vi "Data Buffer Status.vi"(0 "VISA resource name":refnum<visa-resource-name>, 11 "error in (no error)":errorcluster) -> (4 "VISA resource name out":refnum<visa-resource-name>, 6 "Bytes Available":i32, 8 "Bytes in Use":i32, 10 "Next Buffer Location":i32, 15 "error out":errorcluster)   [LabVIEW 2020, in "Keithley 27XX.lvlib"]
doc: "This VI returns information about the status of the buffer including Bytes Available, Bytes in Use, and Next Buffer Location."
uses:
  Keithley 27XX.lvlib
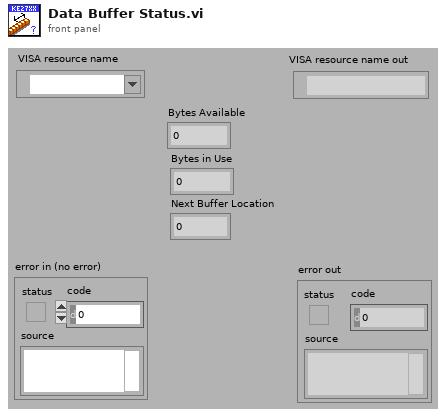
[diagram p1: front panel]
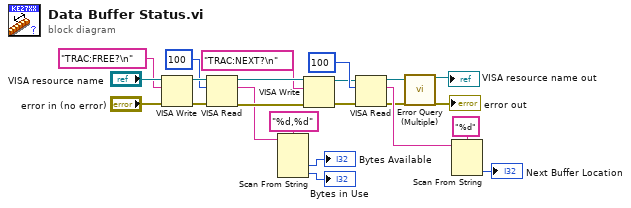
[diagram p0: block diagram]
diagram:
  n1 = VISA Write(VISA resource name="VISA resource name", write buffer="TRAC:FREE?\n", error in (no error)="error in (no error)") -> (VISA resource name out=w19:refnum<visa-resource-name>, error out=w20:errorcluster)  [unwired: 1 out]
  n2 = VISA Read(VISA resource name=w19, byte count=u32 100, error in (no error)=w20) -> (VISA resource name out=w17:refnum<visa-resource-name>, read buffer=w10:string, error out=w16:errorcluster)  [unwired: 1 out]
  n3 = Scan From String(format string="%d,%d", input string=w10) -> (output 1=→"Bytes Available":i32, output 2=→"Bytes in Use":i32)  [unwired: 4 in, 3 out]
  n4 = VISA Write(VISA resource name=w17, write buffer="TRAC:NEXT?\n", error in (no error)=w16) -> (VISA resource name out=w12:refnum<visa-resource-name>, error out=w13:errorcluster)  [unwired: 1 out]
  n5 = VISA Read(VISA resource name=w12, byte count=u32 100, error in (no error)=w13) -> (VISA resource name out=w3:refnum<visa-resource-name>, read buffer=w6:string, error out=w4:errorcluster)  [unwired: 1 out]
  n6 = call "Error Query (Multiple).vi"("VISA resource name"=w3, "error in (no error)"=w4) -> ("VISA resource name out"=→"VISA resource name out":refnum<visa-resource-name>, "error out"=→"error out":errorcluster)  [unwired: 10 in, 2 out]
  n7 = Scan From String(format string="%d", input string=w6) -> (output 1=→"Next Buffer Location":i32)  [unwired: 3 in, 3 out]
